vi "tkrsa6100 Reset.vi"(0 "VISA Resource Name":refnum<visa-resource-name>, 11 "error in (no error)":errorcluster {"code" format="%#.0f"}) -> (4 "dup VISA Resource Name":refnum<visa-resource-name>, 15 "error out":errorcluster {"code" format="%#.0f"})   [LabVIEW 2020, in "Library Instrument & Equipement.lvlib" / "Library Spectrum Analyser.lvlib"]
doc: "This VI executes a *RST command on the instrument.\n\nFirst error in (no error) is checked for any pending errors by tkrsa6100 Write/Read wErrorQuery.vi.\n\nIf error in status is TRUE:\n\nerror in (no error) and VISA Resource Name are passed straight through to error out and dup VISA Resource Name and returned to the calling function. The VI does not execute and no commands are processed.\n\nIf error in status is FALSE:\n\nThe instrument is reset via the *RST command passed to tkrsa6100 Write/Read wErrorQuery.vi. VI input Error Query? of tkrsa6100 Write/Read wErrorQuery.vi is wired to a constant NO since any error query appended to the same line after a *RST would not be executed.\n\nError out is returned to the calling function and VISA Resource Name is returned to the calling function as dup VISA Resource Name."
uses:
  Library Spectrum Analyser.lvlib
panel:
  # "RSA6100 Reset Driver"
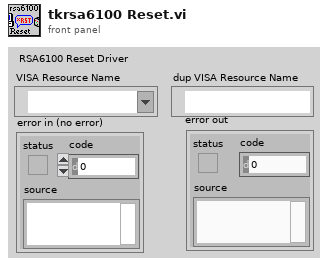
[diagram p1: front panel]
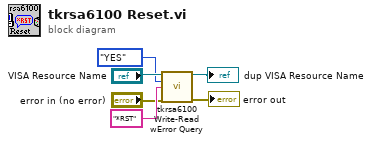
[diagram p0: block diagram]
diagram:
  n1 = call "tkrsa6100 Write-Read wError Query.vi"("VISA Resource Name"="VISA Resource Name", "Error Query(YES)"=enum16{"NO", "YES"}."YES", "Command (Empty String)"="*RST" ("Reset Command"), "error in (no error)"="error in (no error)") -> ("dup VISA Resource Name"=→"dup VISA Resource Name":refnum<visa-resource-name>, "error out"=→"error out":errorcluster)  [unwired: 3 in, 7 out]
